vi "Read Controllable Fullscale Values.vi"(7 "Unit ID (A)":string="A", 8 "error in":errorcluster, 10 "Software Version":u8, 11 "VISA Session In":refnum<visa-resource-name>="Alicat") -> (0 "error out":errorcluster, 2 "Fullscale":T1={"Absolute Pressure"=nan, "Gauge/Diff. Pressure"=nan, "Volumetric Flow"=nan, "Mass Flow"=nan} {"Gauge/Diff. Pressure" format="%_4f"; "Absolute Pressure" format="%_4f"; "Volumetric Flow" format="%_4f"; "Mass Flow" format="%_4f"}, 3 "VISA Session Out":refnum<visa-resource-name>)   [LabVIEW 2024]
doc: "Retrieves fullscale value from device for all controllable measurement types."
uses:
  <vilib>/Instr/_visa.llb/VISA Flush IO Buffer Mask.ctl
panel:
  # "SW Version defaults to 0. \nIf un-wired, it will call a \nsub-VI to check."
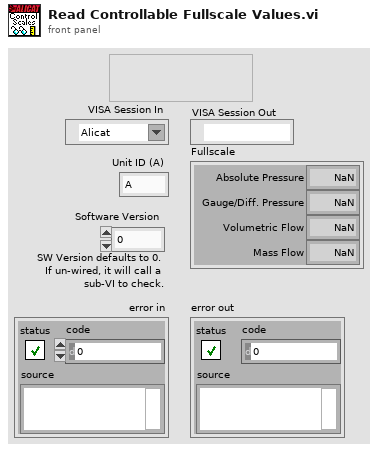
[diagram p1: front panel]
types:
  T1 = cluster{"Absolute Pressure":dbl, "Gauge/Diff. Pressure":dbl, "Volumetric Flow":dbl, "Mass Flow":dbl}
  T2 = cluster{"Pressure":dbl, "Volumetric":dbl, "Mass":dbl}
  T3 = cluster{"Absolute Pressure":dbl, "Gauge/Diff. Pressure":dbl, "Volumetric":dbl, "Mass":dbl}
  T4 = typedef "VISA Flush IO Buffer Mask.ctl" = u16
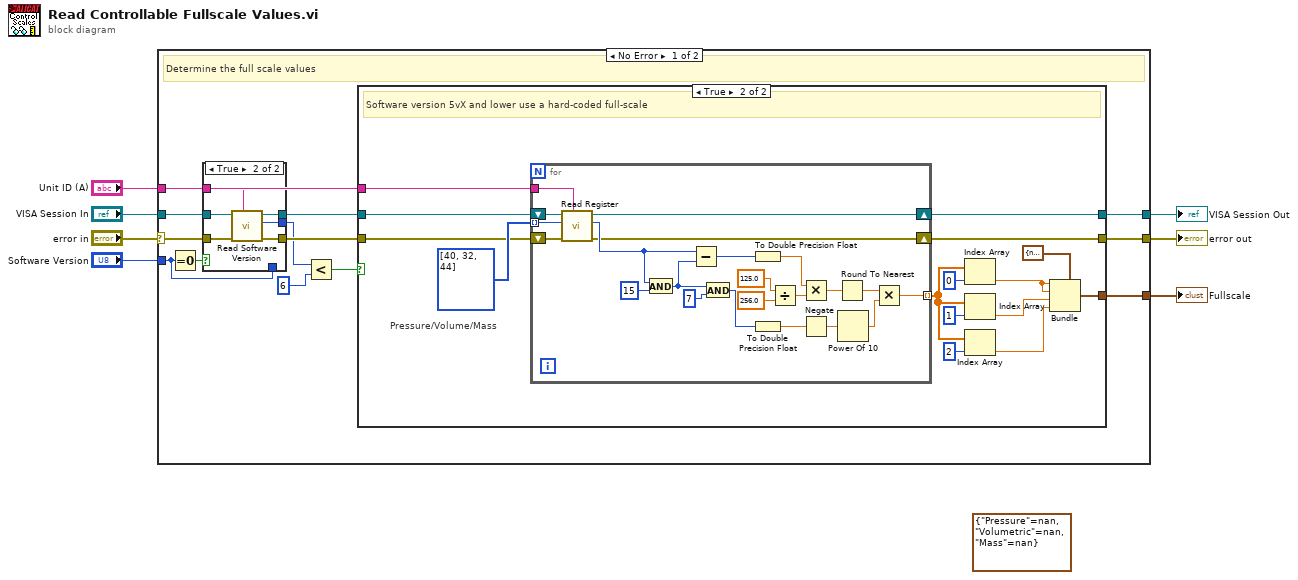
[diagram p0: block diagram]
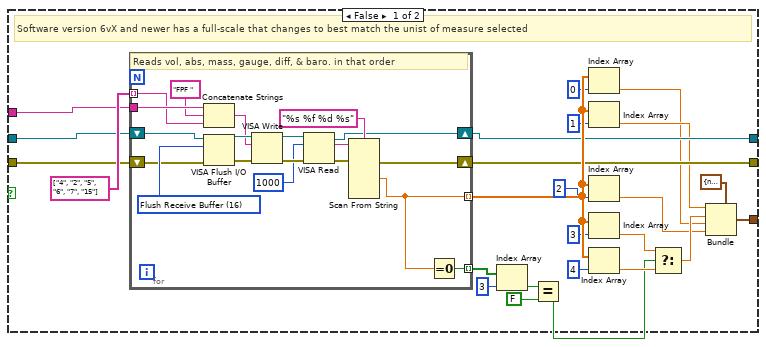
[diagram p2: hidden frame]
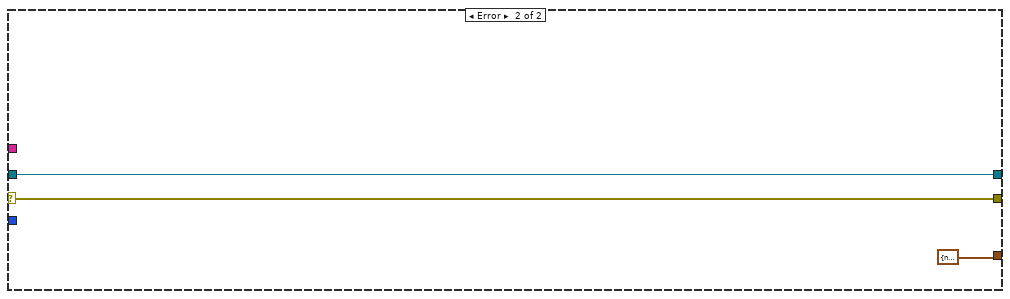
[diagram p4: hidden frame]
diagram:
  (unwired) T2 {"Pressure"=nan, "Volumetric"=nan, "Mass"=nan}
  n1 = case shown="No Error" "error in" {
    selector: "error in" -> [w18 w113]
    tunnel: "VISA Session In" -> [w17 w112]
    tunnel: [w20 w112] -> w6
    tunnel: [w19 w113] -> w5
    tunnel: "Unit ID (A)" -> [w16 _]
    tunnel: [w8 T3 {"Absolute Pressure"=nan, "Gauge/Diff. Pressure"=nan, "Volumetric"=nan, "Mass"=nan} ("Fullscale")] -> w1
    tunnel: "Software Version" -> [w12 _]
    frame No Error {
      # "Determine the full scale values"
      n2 = Equal To 0?(x=w12) -> (x = 0?=w13:bool)
      n3 = case shown="True" w13 {
        tunnel: w18 -> [w103 w110]
        tunnel: w17 -> [w102 w109]
        tunnel: w16 -> [_ w108]
        tunnel: [w103 w107] -> w14
        tunnel: [w102 w106] -> w15
        tunnel: [w104 w105] -> w11
        tunnel: w12 -> [w104 _]
        frame False {
        }
        frame True {
          n4 = call "Read Software Version.vi"("Unit ID (A)"=w108, "error in"=w110, "VISA Session In"=w109) -> ("error out"=w107:errorcluster, "Software Version"=w105:u8, "VISA Session Out"=w106:refnum<visa-resource-name>)  [unwired: 6 in]
        }
      }
      n5 = Less?(x=w11, y=u8 6) -> (x < y?=w9:bool)
      n6 = case shown="True" w9 {
        tunnel: [w27 w79] -> w20
        tunnel: [w28 w78] -> w19
        tunnel: [w24 w65] -> w8
        tunnel: w16 -> [w31 w76]
        tunnel: w15 -> [w30 w75]
        tunnel: w14 -> [w29 w74]
        frame False {
          # "Software version 6vX and newer has a full-scale that changes to best match the unist of measure selected"
          n7 = for {
            tunnel: w31 -> [w54]
            shift-right: [w51] -> w28
            shift-left: w29 -> [w60]
            shift-right: [w50] -> w27
            shift-left: w30 -> [w59]
            tunnel: string[] ["4", "2", "5", "6", "7", "15"] ("appended array") -> [w48] mode=indexing
            tunnel: [w46] -> w38 mode=indexing
            tunnel: [w47] -> w44 mode=indexing
            w63 = T4 16 items=["Flush Receive Buffer"=16, "Write Transmit Buffer to Device"=32, "Flush Receive Buffer (No I/O)"=64, "Flush Transmit Buffer"=128] ("Mask")
            # "Reads vol, abs, mass, gauge, diff, & baro. in that order"
            n8 = Concatenate Strings(w54, "FPF " ("format string (polled)"), w48) -> (w49:string)
            n9 = VISA Flush I/O Buffer(VISA resource name=w59, mask (16)=w63, error in (no error)=w60) -> (VISA resource name out=w56:refnum<visa-resource-name>, error out=w55:errorcluster)
            n10 = VISA Write(VISA resource name=w56, write buffer=w49, error in (no error)=w55) -> (VISA resource name out=w62:refnum<visa-resource-name>, error out=w64:errorcluster)  [unwired: 1 out]
            n11 = VISA Read(VISA resource name=w62, byte count=u32 1000, error in (no error)=w64) -> (VISA resource name out=w50:refnum<visa-resource-name>, read buffer=w57:string, error out=w52:errorcluster)  [unwired: 1 out]
            n12 = Scan From String(format string="%s %f %d %s", input string=w57, error in=w52) -> (error out=w51:errorcluster, output 2=w46:dbl)  [unwired: 8 in, 2 out]
            n13 = Equal To 0?(x=w46) -> (x = 0?=w47:bool)
          }
          n14 = Index Array(array=w44, index=3) -> (element=w42:bool)
          n15 = Equal?(x=w42, y=FALSE) -> (x = y?=w32:bool)
          n16 = Index Array(array=w38, index=0) -> (element=w22:dbl)
          n17 = Index Array(array=w38, index=1) -> (element=w26:dbl)
          n18 = Index Array(array=w38, index=2) -> (element=w21:dbl)
          n19 = Index Array(array=w38, index=3) -> (element=w40:dbl)
          n20 = Index Array(array=w38, index=4) -> (element=w39:dbl)
          n21 = Select(t=w40, s=w32, f=w39) -> (s? t:f=w25:dbl)
          n22 = Bundle(cluster=T3 {"Absolute Pressure"=nan, "Gauge/Diff. Pressure"=nan, "Volumetric"=nan, "Mass"=nan} ("Fullscale"), "Absolute Pressure"=w26, "Gauge/Diff. Pressure"=w25, "Volumetric"=w22, "Mass"=w21) -> (w24:T3)
        }
        frame True {
          # "Pressure/Volume/Mass"
          # "Software version 5vX and lower use a hard-coded full-scale"
          n23 = for {
            tunnel: [w100] -> w73 mode=indexing
            tunnel: u16[] [40, 32, 44] -> [w99] mode=indexing
            tunnel: w76 -> [w94]
            shift-right: [w96] -> w79
            shift-left: w75 -> [w97]
            shift-right: [w95] -> w78
            shift-left: w74 -> [w98]
            n24 = call "Read Register.vi"("Unit ID (A)"=w94, "error in"=w98, "Register address"=w99, "VISA Session In"=w97) -> ("error out"=w95:errorcluster, "Register Value (I32)"=w101:i32, "VISA Session Out"=w96:refnum<visa-resource-name>)  [unwired: 5 in]
            n25 = And(x=w101, y=15) -> (x .and. y?=w86:i32)
            n26 = Subtract(x=w101, y=w86) -> (x-y=w83:i32)
            n27 = And(x=w86, y=7) -> (x .and. y?=w90:i32)
            n28 = To Double Precision Float(number=w83) -> (double precision float=w84:dbl)
            n29 = To Double Precision Float(number=w90) -> (double precision float=w89:dbl)
            n30 = Divide(x=125.0 ("y"), y=256.0) -> (x/y=w85:dbl)
            n31 = Multiply(x=w84, y=w85) -> (x*y=w92:dbl)
            n32 = Negate(x=w89) -> (-x=w88:dbl)
            n33 = Round To Nearest(number=w92) -> (nearest integer value=w93:dbl)
            n34 = Power Of 10(x=w88) -> (10^x=w91:dbl)
            n35 = Multiply(x=w93, y=w91) -> (x*y=w100:dbl)
          }
          n36 = Index Array(array=w73, index=0) -> (element=w69:dbl)
          n37 = Index Array(array=w73, index=1) -> (element=w67:dbl)
          n38 = Index Array(array=w73, index=2) -> (element=w66:dbl)
          n39 = Bundle(cluster=T3 {"Absolute Pressure"=nan, "Gauge/Diff. Pressure"=nan, "Volumetric"=nan, "Mass"=nan} ("Fullscale"), "Absolute Pressure"=w69, "Gauge/Diff. Pressure"=w69, "Volumetric"=w67, "Mass"=w66) -> (w65:T3)
        }
      }
    }
    frame Error {
    }
  }
  "error out" <- w5
  "VISA Session Out" <- w6
  "Fullscale" <- w1
